vi "mqttTCPIPserver.vi"(0 "mqtt.lvclass":refnum<class "mqtt.lvclass">, 11 "error in (no error)":errorcluster) -> (4 "mqtt.lvclass 2":refnum<class "mqtt.lvclass">, 15 "error out":errorcluster)   [LabVIEW 2017, in "mqtt.lvclass"]
uses:
  mqtt.lvclass
  mqttTXqueue/mqttTXdataQueueFunction.ctl
  mqtt.lvclass/mqtt.ctl
  mqttTypedef/mqttRXdataCluster.ctl
  mqttTypedef/mqttFixedHeaderResponse.ctl
  mqttTypedef/mqttQOSlevel.ctl
  mqttTypedef/mqttMessageType.ctl
  mqttTXqueue/mqttRXsubscriptionEventFunction.ctl
  mqttTXqueue/mqttRXsubscriptionEventData.ctl
panel:
  out "exit signal":bool
  in  "outer loop":bool=TRUE
  out "error out 3":errorcluster
  out "error out 2":errorcluster
  out "rxCount":i32
  out "rxTelegram":u8[](array[numeric]) format="%02x"
  out "txError":errorcluster
  out "txTelegram":u8[](array[numeric]) format="%02x"
  out "payloadError":errorcluster
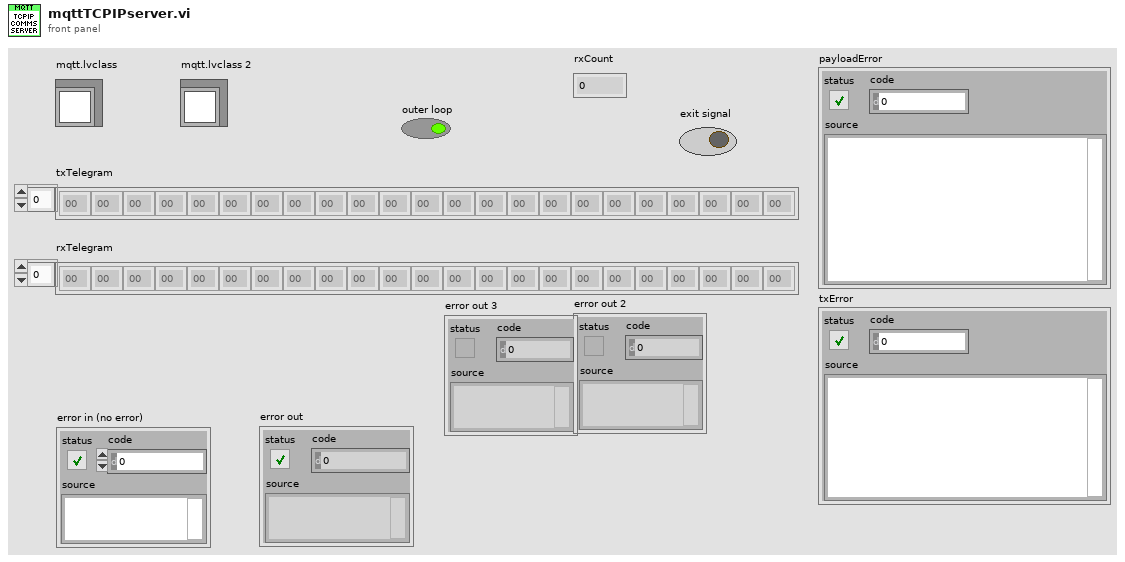
[diagram p1: front panel]
types:
  T1 = typedef "mqttTXdataQueueFunction.ctl" = enum16{"init", "deinit", "getQueue", "enqueue"}
  T2 = typedef "mqttRXdataCluster.ctl" = cluster{"fixedHdr":T3, "payload":u8[]}
  T3 = typedef "mqttFixedHeaderResponse.ctl" = cluster{"retain":bool, "qos":T4, "duplicate":bool, "response":T5}
  T4 = typedef "mqttQOSlevel.ctl" = enum8{"At most once", "At least once", "Exactly once", "Reserved"}
  T5 = typedef "mqttMessageType.ctl" = enum32{"Reserved", "CONNECT", "CONNACK", "PUBLISH", "PUBACK", "PUBREC", "PUBREL", "PUBCOMP", "SUBSCRIBE", "SUBACK", "UNSUBSCRIBE", "UNSUBACK", "PINGREQ", "PINGRESP", "DISCONNECT", "Reserved2"}
  T6 = typedef "mqttRXsubscriptionEventData.ctl" = cluster{"topic":string, "value":string, "messageID":u16}
  T7 = typedef "mqttRXsubscriptionEventFunction.ctl" = enum16{"init", "deinit", "getEventRef", "event"}
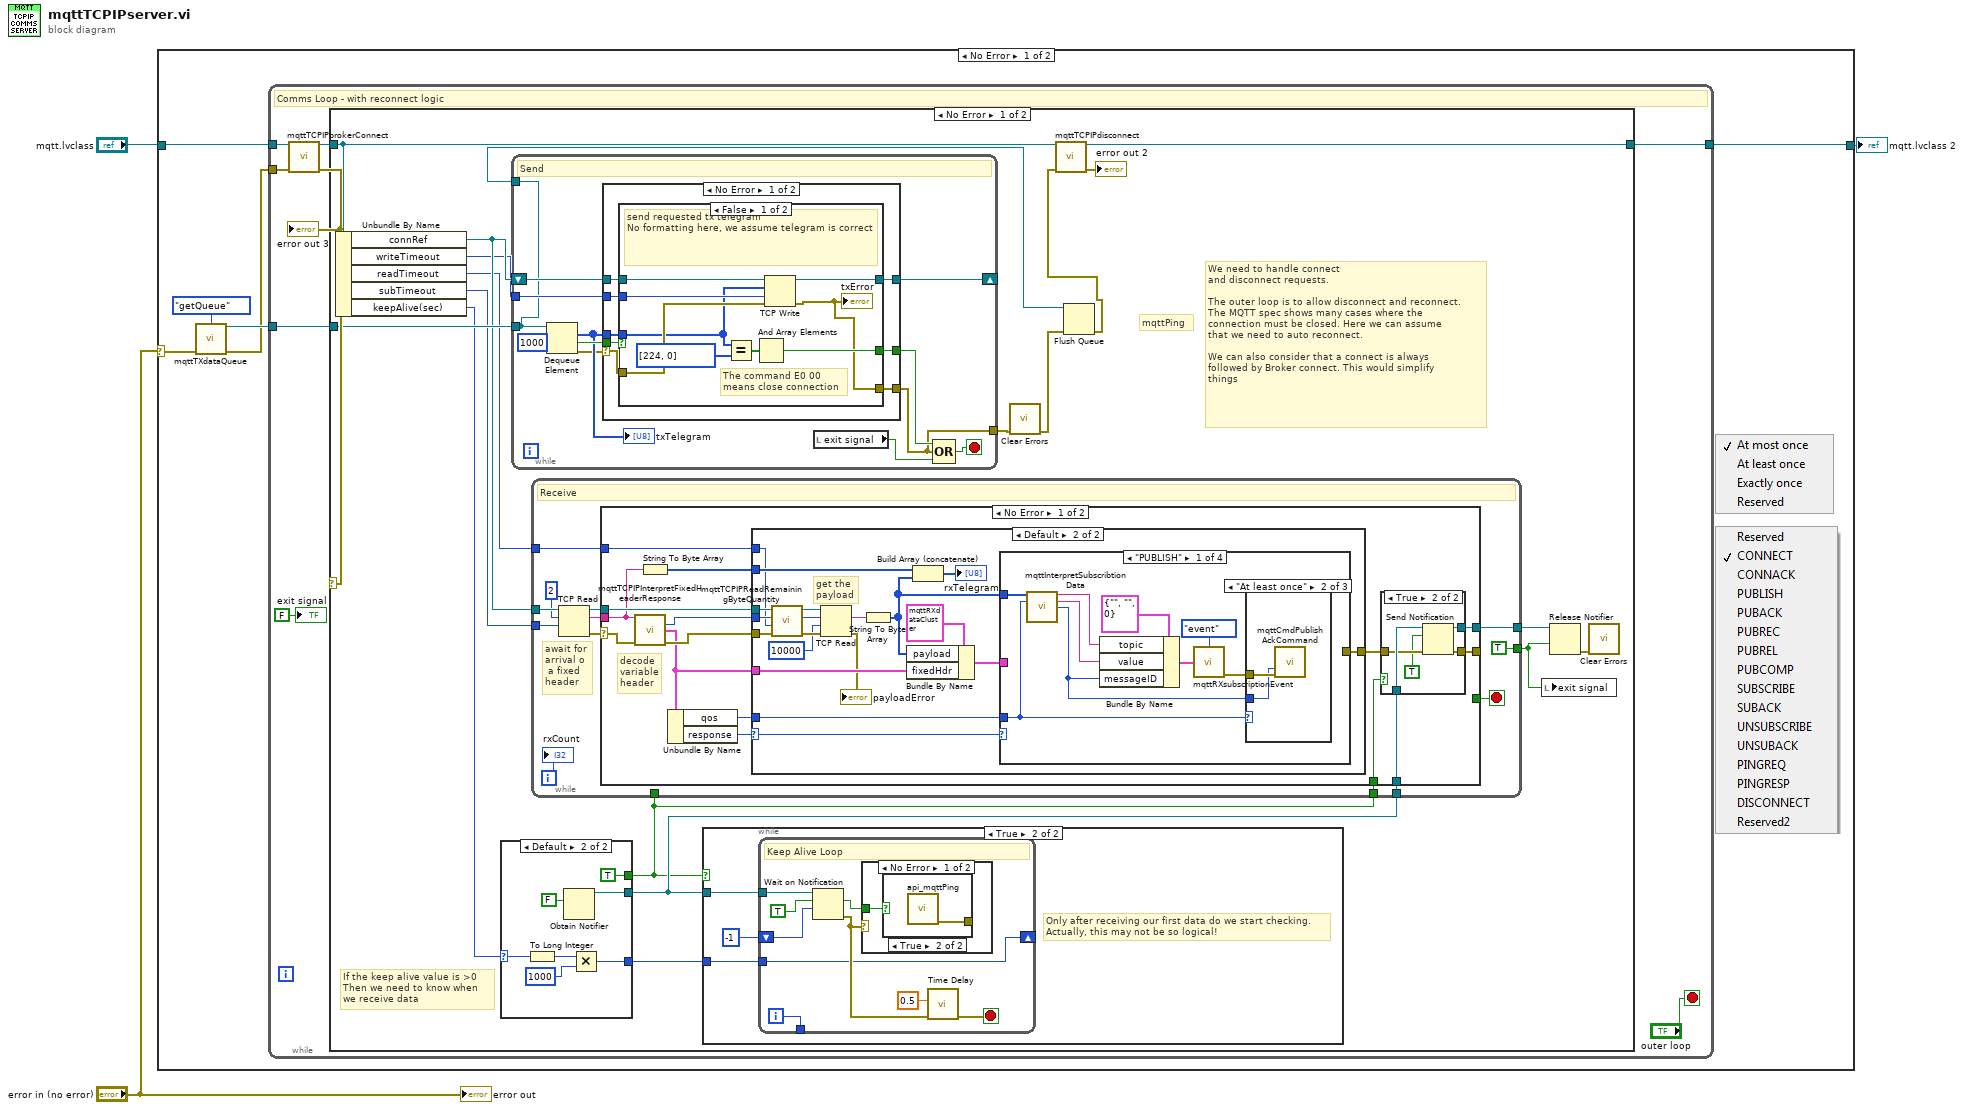
[diagram p0: block diagram]
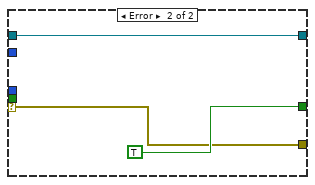
[diagram p7: hidden frame]
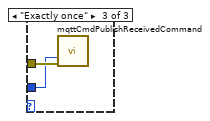
[diagram p11: hidden frame]
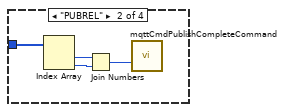
[diagram p12: hidden frame]
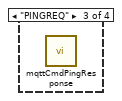
[diagram p13: hidden frame]
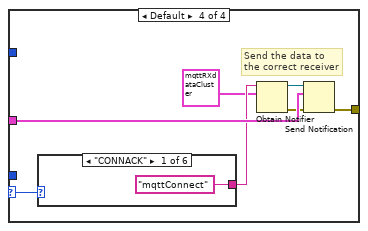
[diagram p14: hidden frame]
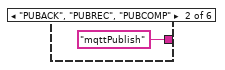
[diagram p15: hidden frame]
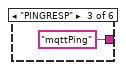
[diagram p16: hidden frame]
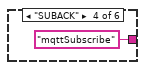
[diagram p17: hidden frame]
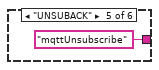
[diagram p18: hidden frame]
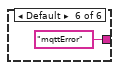
[diagram p19: hidden frame]
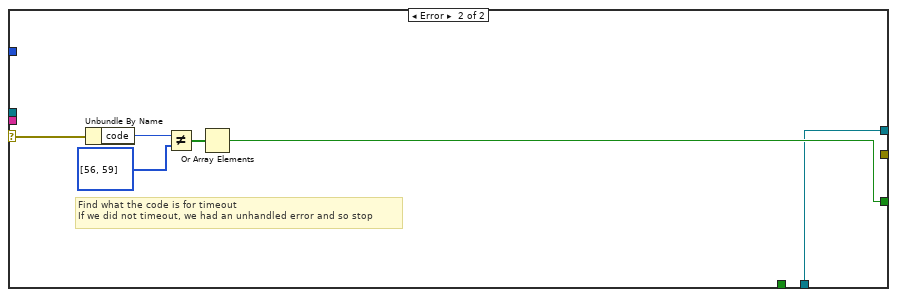
[diagram p20: hidden frame]
diagram:
  n1 = case shown="No Error" "error in (no error)" {
    selector: "error in (no error)" -> [w4 _]
    tunnel: "mqtt.lvclass" -> [w7 w181]
    tunnel: [w6 w181] -> w2
    frame No Error {
      n2 = call "mqttTXdataQueue.vi"("function"=mqttTXdataQueueFunction."getQueue", "error in (no error)"=w4) -> ("Queue out"=w9:refnum<queue>, "error out"=w5:errorcluster)  [unwired: 12 in]
      n3 = while {
        tunnel: w9 -> [w17]
        tunnel: w7 -> [w15]
        tunnel: [w13] -> w6
        tunnel: w5 -> [w14]
        stop <- "outer loop" stop-if-true
        # "Comms Loop - with reconnect logic"
        n4 = call "mqttTCPIPbrokerConnect.vi"("mqtt in"=w15, "error in (no error)"=w14) -> ("mqtt out"=w12:refnum<class "mqtt.lvclass">, "error out"=w11:errorcluster)  [unwired: 12 in]
        "error out 3" <- w11
        n5 = case shown="No Error" w11 {
          tunnel: w17 -> [w36 _]
          tunnel: [w33 w180] -> w13
          tunnel: w12 -> [w32 w180]
          frame No Error {
            # "If the keep alive value is >0\nThen we need to know when\nwe receive data"
            # "mqttPing"
            # "We need to handle connect\nand disconnect requests.\n\nThe outer loop is to allow disconnect and reconnect.\nThe MQTT spec shows many cases where the\nconnection must be closed. Here we can assume\nthat we need to auto reconnect.\n\nWe can also consider that a connect is always\nfollowed by Broker connect. This would simplify\nthings"
            n6 = Unbundle By Name(w32) -> ("connRef"=w35:refnum<k5>, "writeTimeout"=w31:i32, "readTimeout"=w30:i32, "subTimeout"=w29:i32, "keepAlive(sec)"=w24:u16)
            n7 = case shown="Default" w24 {
              selector: w24 -> [_ w52]
              tunnel: [_ w57] -> w28
              tunnel: [_ w53] -> w25
              tunnel: [_ TRUE] -> w23
              frame ..0 {
              }
              frame Default {
                n8 = To Long Integer(number=w52) -> (32bit integer=w55:i32)
                n9 = Obtain Notifier(notification data type=FALSE) -> (notifier out=w57:refnum<notifier>)  [unwired: 3 in, 2 out]
                n10 = Multiply(x=w55, y=1000) -> (x*y=w53:i32)
              }
            }
            n11 = while {
              tunnel: w36 -> [w59]
              shift-right: [w67] -> _
              shift-left: w35 -> [w68]
              tunnel: [w61] -> w34
              tunnel: w31 -> [w63]
              tunnel: [w59] -> w21
              stop <- w66 stop-if-true
              # "Send"
              n12 = Dequeue Element(queue=w59, timeout in ms (-1)=1000) -> (element=w64:u8[], timed out?=w69:bool, error out=w62:errorcluster)  [unwired: 1 in, 1 out]
              "txTelegram" <- w64
              n13 = case shown="No Error" w62 {
                selector: w62 -> [w71 w89]
                tunnel: w69 -> [w77 _]
                tunnel: w64 -> [w76 _]
                tunnel: w68 -> [w75 w91]
                tunnel: [w74 w91] -> w67
                tunnel: [w73 TRUE] -> w65
                tunnel: w63 -> [w72 _]
                tunnel: [w70 w89] -> w61
                frame No Error {
                  n14 = case shown="False" w77 {
                    tunnel: w76 -> [w78 _]
                    tunnel: w75 -> [w86 w88]
                    tunnel: [w85 w88] -> w74
                    tunnel: [w82 _] -> w73
                    tunnel: w72 -> [w81 _]
                    tunnel: w71 -> [w80 w87]
                    tunnel: [w79 w87] -> w70
                    frame False {
                      # "The command E0 00\nmeans close connection"
                      # "send requested tx telegram\nNo formatting here, we assume telegram is correct"
                      n15 = Equal?(x=w78, y=u8[] [224, 0] ("txTelegram 2")) -> (x = y?=w83:bool[])
                      n16 = And Array Elements(Boolean array=w83) -> (logical AND=w82:bool)
                      n17 = TCP Write(connection ID=w86, data in=w78, error in (no error)=w80, 9:w81) -> (connection ID out=w85:refnum<k5>, error out=w79:errorcluster)  [unwired: 1 out]
                      "txError" <- w79
                    }
                    frame True {
                      # "Queue Timed Out - do nothing.\nWe can later use this for the Keep Alive ping"
                    }
                  }
                }
                frame Error {
                }
              }
              n18 = local read "exit signal"() -> (w58:bool)
              n19 = Compound Arithmetic op=OR(w65, w61, w58) -> (w66:bool)
            }
            n20 = while {
              tunnel: w35 -> [w104]
              tunnel: w30 -> [w97]
              tunnel: w29 -> [w96]
              tunnel: w28 -> [w95]
              tunnel: [w94] -> w27
              tunnel: w23 -> [w93]
              tunnel: w23 -> [_]
              tunnel: [TRUE ("force destroy? (F)")] -> w18
              i -> [w98]
              stop <- w99 stop-if-true
              # "await for\narrival o\n a fixed\nheader"
              # "Receive"
              n21 = TCP Read(connection ID=w104, bytes to read=2, 9:w96) -> (connection ID out=w103:refnum<k5>, data out=w100:string, error out=w102:errorcluster)  [unwired: 2 in]
              n22 = case shown="No Error" w102 {
                selector: w102 -> [w117 w179]
                tunnel: w103 -> [w118 _]
                tunnel: w100 -> [w113 _]
                tunnel: [_ w175] -> w99
                tunnel: w97 -> [w110 _]
                tunnel: w95 -> [w109 w174]
                tunnel: [w107 w174] -> w94
                tunnel: [w106 _] -> _
                tunnel: w93 -> [w105 _]
                frame No Error {
                  # "decode\nvariable\nheader"
                  n23 = call "mqttTCPIPInterpretFixedHeaderResponse.vi"("data in"=w113, "error in (no error)"=w117) -> ("remainingLengthByte1"=w119:u8, "output cluster"=w115:T3, "error out"=w116:errorcluster)  [unwired: 11 in]
                  n24 = String To Byte Array(string=w113) -> (unsigned byte array=w112:u8[])
                  n25 = Unbundle By Name(w115) -> ("qos"=w111:T4, "response"=w114:T5)
                  n26 = case shown="Default" w114 {
                    selector: w114 -> [_ w133]
                    tunnel: w119 -> [_ w143]
                    tunnel: w118 -> [_ w142]
                    tunnel: w116 -> [_ w135]
                    tunnel: w115 -> [_ w134]
                    tunnel: w112 -> [_ w130]
                    tunnel: w111 -> [_ w129]
                    tunnel: w110 -> [_ w126]
                    tunnel: [_ w125] -> w108
                    frame "CONNECT", "SUBSCRIBE" {
                      # "The client should not receive these commands.\nI had some problems with these commands being received\nand it appears this was a broker issue. However, to ignore\nmessages that we should not receive is no bad thing."
                    }
                    frame Default {
                      # "get the\npayload"
                      n27 = call "mqttTCPIPReadRemainingByteQuantity.vi"("error in (no error)"=w135, "readTimeout ms (2000)"=w126, "remainingLengthByte1"=w143, "connRef in"=w142) -> ("error out"=w140:errorcluster, "remainingLength"=w139:i32, "connRef out"=w141:refnum<k5>)  [unwired: 5 in]
                      n28 = TCP Read(connection ID=w141, bytes to read=w139, error in (no error)=w140, 9:10000 ("timeout ms (25000)")) -> (data out=w137:string, error out=→"payloadError":errorcluster)  [unwired: 1 in, 1 out]
                      n29 = String To Byte Array(string=w137) -> (unsigned byte array=w127:u8[])
                      n30 = Bundle By Name(cluster=T2 {"fixedHdr"={"retain"=FALSE, "qos"=enum."At most once", "duplicate"=FALSE, "response"=enum."Reserved"}, "payload"=[]} ("output cluster"), "payload"=w127, "fixedHdr"=w134) -> (w131:T2)
                      n31 = Build Array (concatenate)(w130, w127) -> (→"rxTelegram":u8[])
                      n32 = case shown="\"PUBLISH\"" w133 {
                        selector: w133 -> [_ _ _ w167]
                        tunnel: w131 -> [_ _ _ w166]
                        tunnel: w129 -> [w145 _ _ _]
                        tunnel: w127 -> [w149 w160 _ _]
                        tunnel: [_ _ _ w161] -> w125
                        frame "PUBLISH" {
                          n33 = call "mqttInterpretSubscribtionData.vi"("rxTelegram in"=w149, "qos"=w145) -> ("topic"=w148:string, "value"=w147:string, "messageID"=w144:u16)  [unwired: 10 in, 1 out]
                          n34 = Bundle By Name(cluster=T6 {"topic"="", "value"="", "messageID"=0} ("data"), "topic"=w148, "value"=w147, "messageID"=w144) -> (w150:T6)
                          n35 = call "mqttRXsubscriptionEvent.vi"("function"=mqttRXsubscriptionEventFunction."event", "data"=w150) -> ("error out"=w146:errorcluster)  [unwired: 12 in, 1 out]
                          n36 = case shown="\"At least once\"" w145 {
                            tunnel: w146 -> [_ w154 w156]
                            tunnel: w144 -> [_ w153 w155]
                            frame Default {
                            }
                            frame "At least once" {
                              n37 = call "mqttCmdPublishAckCommand.vi"("messageID"=w153, "error in (no error)"=w154) -> ()  [unwired: 13 in, 1 out]
                            }
                            frame "Exactly once" {
                              n38 = call "mqttCmdPublishReceivedCommand.vi"("messageID"=w155, "error in (no error)"=w156) -> ()  [unwired: 13 in, 1 out]
                            }
                          }
                        }
                        frame "PUBREL" {
                          n39 = Index Array(array=w160) -> (element #1=w159:u8, element #2=w158:u8)  [unwired: 2 in]
                          n40 = Join Numbers(hi=w159, lo=w158) -> ((hi.lo)=w157:u16)
                          n41 = call "mqttCmdPublishCompleteCommand.vi"("messageID"=w157) -> ()  [unwired: 14 in, 1 out]
                        }
                        frame "PINGREQ" {
                          n42 = call "mqttCmdPingResponse.vi"() -> ()  [unwired: 15 in, 1 out]
                        }
                        frame Default {
                          # "Send the data to\nthe correct receiver"
                          n43 = case shown="\"CONNACK\"" w167 {
                            tunnel: ["mqttConnect" ("name (unnamed)") "mqttPublish" ("name (unnamed)") "mqttPing" ("name (unnamed)") "mqttSubscribe" ("name (unnamed)") "mqttUnsubscribe" ("name (unnamed)") "mqttError" ("name (unnamed)")] -> w165
                            frame "CONNACK" {
                            }
                            frame "PUBACK", "PUBREC", "PUBCOMP" {
                            }
                            frame "PINGRESP" {
                            }
                            frame "SUBACK" {
                            }
                            frame "UNSUBACK" {
                            }
                            frame Default {
                            }
                          }
                          n44 = Obtain Notifier(name (unnamed)=w165, notification data type=T2 {"fixedHdr"={"retain"=FALSE, "qos"=enum."At most once", "duplicate"=FALSE, "response"=enum."Reserved"}, "payload"=[]} ("output cluster")) -> (notifier out=w164:refnum<notifier>, error out=w162:errorcluster)  [unwired: 2 in, 1 out]
                          n45 = Send Notification(notification=w166, notifier=w164, error in (no error)=w162) -> (error out=w161:errorcluster)  [unwired: 1 out]
                        }
                      }
                    }
                  }
                  n46 = case shown="True" w105 {
                    tunnel: w109 -> [_ w124]
                    tunnel: w108 -> [_ w123]
                    tunnel: [_ w121] -> w107
                    tunnel: [_ w120] -> w106
                    frame False {
                    }
                    frame True {
                      n47 = Send Notification(notification=TRUE, notifier=w124, error in (no error)=w123) -> (notifier out=w121:refnum<notifier>, error out=w120:errorcluster)
                    }
                  }
                }
                frame Error {
                  # "Find what the code is for timeout\nIf we did not timeout, we had an unhandled error and so stop"
                  n48 = Unbundle By Name(w179) -> ("code"=w178:i32)
                  n49 = Not Equal?(x=w178, y=i32[] [56, 59]) -> (x != y?=w176:bool[])
                  n50 = Or Array Elements(Boolean array=w176) -> (logical OR=w175:bool)
                }
              }
              "rxCount" <- w98
            }
            n51 = case shown="True" w23 {
              tunnel: w28 -> [_ w39]
              tunnel: w25 -> [_ w38]
              frame False {
              }
              frame True {
                # "Only after receiving our first data do we start checking.\nActually, this may not be so logical!"
                n52 = while {
                  tunnel: w39 -> [w48]
                  tunnel: [w44] -> _
                  shift-right: [w41] -> _
                  shift-left: -1 -> [w47]
                  tunnel: w38 -> [w41]
                  i -> [w44]
                  stop <- w45 stop-if-true
                  # "Keep Alive Loop"
                  n53 = Wait on Notification(notifier=w48, ignore previous (F)=TRUE, timeout in ms (-1)=w47) -> (notification=w40:bool, error out=w42:errorcluster)  [unwired: 1 in, 2 out]
                  n54 = case shown="No Error" w42 {
                    tunnel: w40 -> [w49 _]
                    frame No Error {
                      n55 = case shown="True" w49 {
                        tunnel: [_ w50] -> _
                        frame False {
                        }
                        frame True {
                          n56 = call "api_mqttPing.vi"() -> ("error out"=w50:errorcluster)  [unwired: 14 in, 1 out]
                        }
                      }
                    }
                    frame Error {
                    }
                  }
                  n57 = call "Time Delay"("error in (no error)"=w42, "Delay Time (s)"=0.5) -> ("error out"=w45:errorcluster)  [unwired: 9 in]
                }
              }
            }
            n58 = call <vilib>:"Clear Errors.vi"("error in (no error)"=w34) -> ("error out"=w20:errorcluster)  [unwired: 5 in, 1 out]
            n59 = Flush Queue(queue=w21, error in (no error)=w20) -> (error out=w19:errorcluster)  [unwired: 2 out]
            n60 = call "mqttTCPIPdisconnect.vi"("mqtt in"=w32, "error in (no error)"=w19) -> ("mqtt out"=w33:refnum<class "mqtt.lvclass">, "error out"=→"error out 2":errorcluster)  [unwired: 12 in]
            n61 = local write "exit signal"(w18) -> ()
            n62 = Release Notifier(notifier=w27, force destroy? (F)=w18) -> (error out=w26:errorcluster)  [unwired: 1 in, 2 out]
            n63 = call <vilib>:"Clear Errors.vi"("error in (no error)"=w26) -> ()  [unwired: 5 in, 2 out]
          }
          frame Error {
            # "Doesn't make sense to do stuff if there is no TCP connection"
          }
        }
        "exit signal" <- FALSE ("exit signal")
      }
    }
    frame Error {
    }
  }
  "mqtt.lvclass 2" <- w2
  "error out" <- "error in (no error)"
